vi "摩擦力F.vi"(8 "计算参数 in":T2, 9 "输入参数":T1, 10 "进油口压力数组 in":dbl[](array[numeric]), 11 "行程数组 in":dbl[](array[numeric])) -> (0 "计算参数 out":T2, 2 "进油口压力数组 out":dbl[](array[numeric]), 3 "行程数组 out":dbl[](array[numeric]))   [LabVIEW 2013]
doc: "此程序计算开启关闭时间\nCL=tv2-tv1\nOP=ts2-ts1"
panel:
  out "P":dbl[](array[numeric])
  out "TIME_DOWN":dbl[](array[numeric])
  out "TIME_UP":dbl[](array[numeric])
  out "V":dbl[](array[numeric])
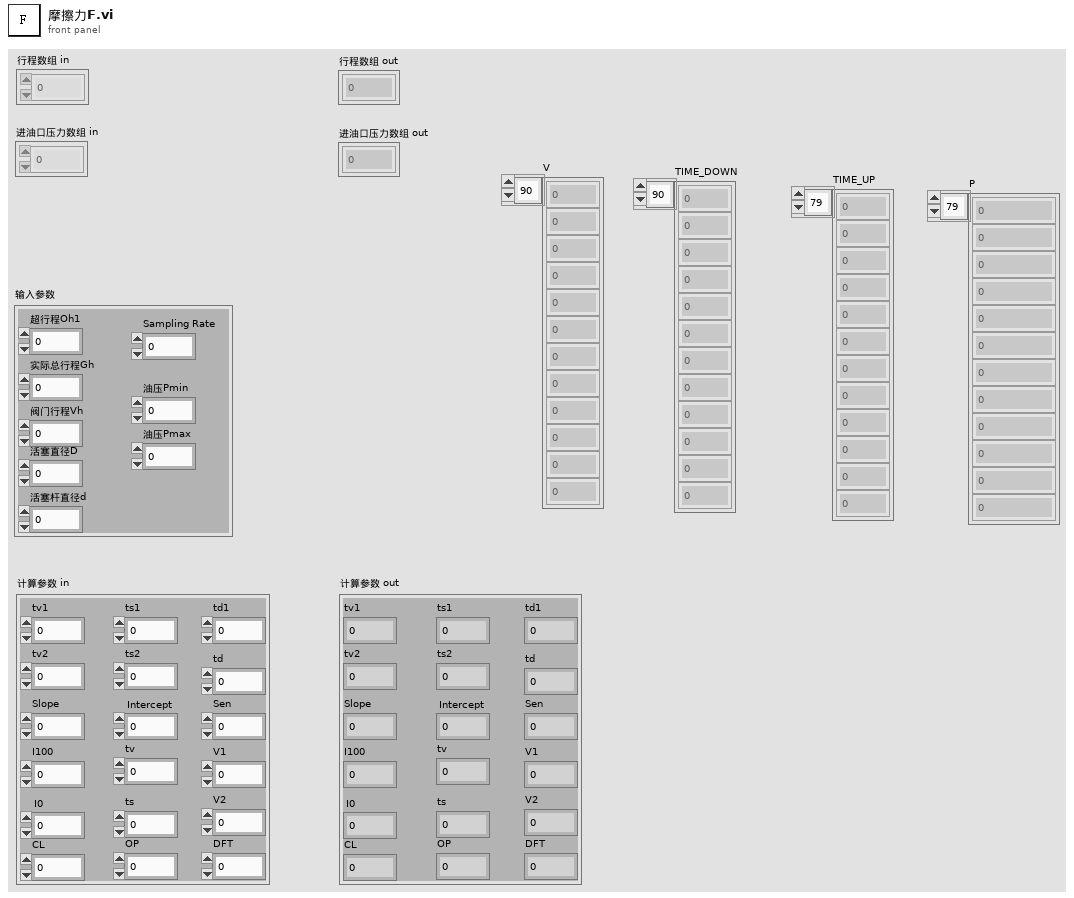
[diagram p1: front panel]
types:
  T1 = cluster{"超行程Oh1":dbl, "实际总行程Gh":dbl, "阀门行程Vh":dbl, "活塞直径D":dbl, "活塞杆直径d":dbl, "油压Pmin":dbl, "油压Pmax":dbl, "Sampling Rate":dbl}
  T2 = cluster{"tv1":dbl, "tv2":dbl, "tv":dbl, "ts1":dbl, "ts2":dbl, "ts":dbl, "td1":dbl, "td":dbl, "Slope":dbl, "Intercept":dbl, "I100":dbl, "I0":dbl, "Sen":dbl, "V1":dbl, "V2":dbl, "CL":dbl, "OP":dbl, "DFT":dbl}
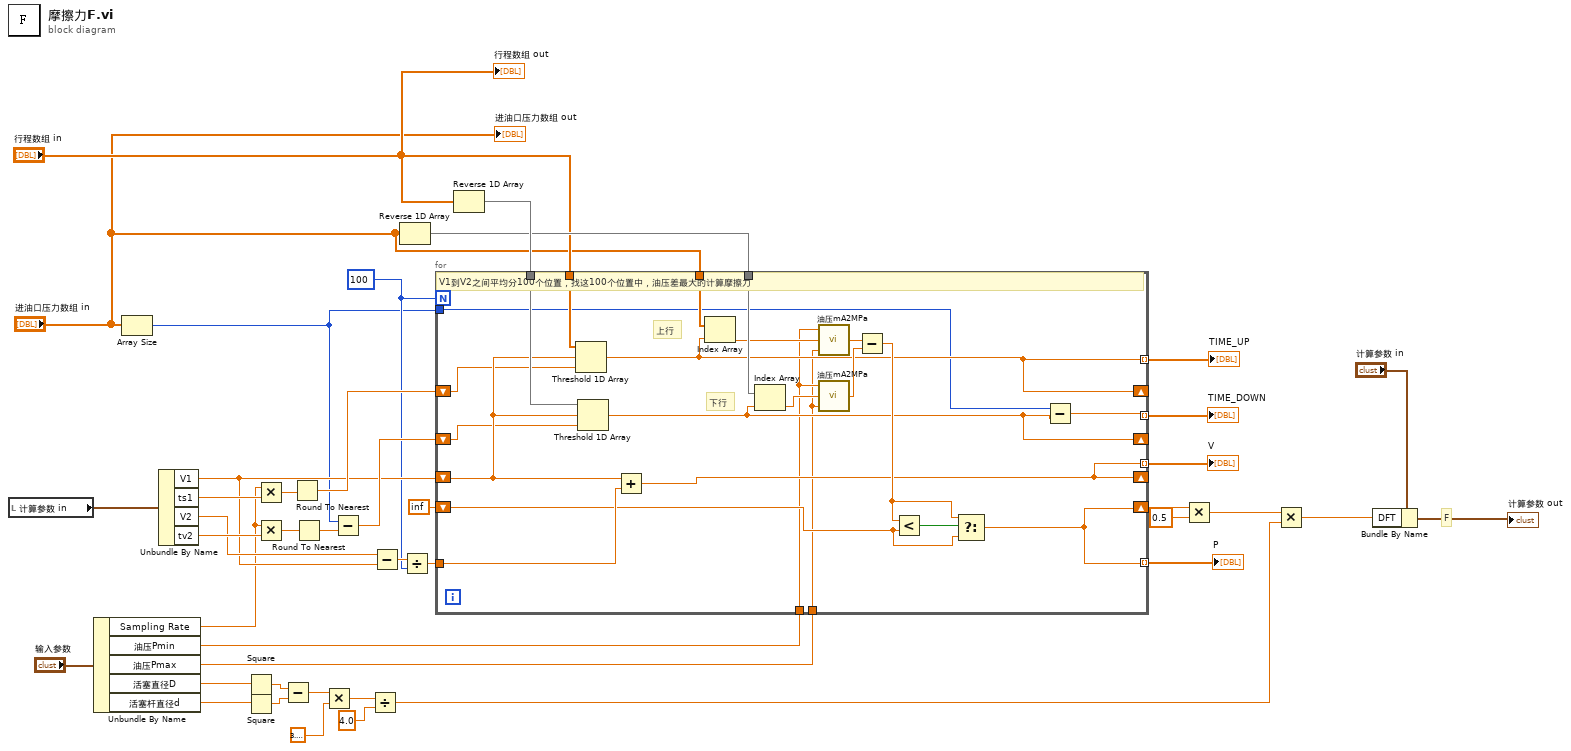
[diagram p0: block diagram]
diagram:
  w20 = 100
  # "F"
  n1 = local read "计算参数 in"() -> (w40:T2)
  n2 = Unbundle By Name("输入参数") -> ("Sampling Rate"=w1:dbl, "油压Pmin"=w3:dbl, "油压Pmax"=w2:dbl, "活塞直径D"=w38:dbl, "活塞杆直径d"=w37:dbl)
  n3 = Array Size(array="进油口压力数组 in") -> (size(s)=w5:i32)
  n4 = Unbundle By Name(w40) -> ("V1"=w22:dbl, "ts1"=w29:dbl, "V2"=w23:dbl, "tv2"=w27:dbl)
  n5 = Square(x=w38) -> (x^2=w36:dbl)
  n6 = Square(x=w37) -> (x^2=w35:dbl)
  n7 = Multiply(x=w1, y=w29) -> (x*y=w30:dbl)
  n8 = Multiply(x=w1, y=w27) -> (x*y=w28:dbl)
  n9 = Subtract(x=w36, y=w35) -> (x-y=w34:dbl)
  n10 = Round To Nearest(number=w30) -> (nearest integer value=w25:dbl)
  n11 = Round To Nearest(number=w28) -> (nearest integer value=w26:dbl)
  n12 = Multiply(x=w34, y=3.141592653589793) -> (x*y=w32:dbl)
  n13 = Subtract(x=w5, y=w26) -> (x-y=w24:dbl)
  n14 = Divide(x=w32, y=4.0) -> (x/y=w13:dbl)
  n15 = Subtract(x=w23, y=w22) -> (x-y=w21:dbl)
  n16 = Reverse 1D Array(array="进油口压力数组 in") -> (reversed array=w16:dbl[])
  n17 = Divide(x=w21, y=w20) -> (x/y=w19:dbl)
  n18 = Reverse 1D Array(array="行程数组 in") -> (reversed array=w17:dbl[])
  n19 = for {
    N: w20 -> [_]
    shift-right: [w49] -> _
    shift-left: w25 -> [w60]
    shift-right: [w47] -> _
    shift-left: w24 -> [w61]
    tunnel: "行程数组 in" -> [w65]
    shift-right: [w50] -> _
    shift-left: w22 -> [w62]
    tunnel: w19 -> [w64]
    shift-right: [w45] -> w15
    shift-left: inf -> [w56]
    tunnel: w17 -> [w63]
    tunnel: w16 -> [w59]
    tunnel: "进油口压力数组 in" -> [w58]
    tunnel: [w50] -> w8 mode=indexing
    tunnel: [w49] -> w7 mode=indexing
    tunnel: [w48] -> w6 mode=indexing
    tunnel: w5 -> [w46]
    tunnel: [w45] -> w4 mode=indexing
    tunnel: w3 -> [w44]
    tunnel: w2 -> [w43]
    # "下行"
    # "上行"
    # "V1到V2之间平均分100个位置，找这100个位置中，油压差最大的计算摩擦力"
    n20 = Threshold 1D Array(1:w60, 2:w62, 3:w65) -> (0:w49:dbl)
    n21 = Threshold 1D Array(1:w61, 2:w62, 3:w63) -> (0:w47:dbl)
    n22 = Add(x=w62, y=w64) -> (x+y=w50:dbl)
    n23 = Index Array(array=w58, index=w49) -> (element=w53:dbl)
    n24 = Index Array(array=w59, index=w47) -> (element=w52:dbl)
    n25 = call "油压mA2MPa.vi"("油压Max"=w43, "油压mA"=w53, "油压Min"=w44) -> ("油压MPa"=w54:dbl)  [unwired: 2 in]
    n26 = call "油压mA2MPa.vi"("油压Max"=w43, "油压mA"=w52, "油压Min"=w44) -> ("油压MPa"=w51:dbl)  [unwired: 2 in]
    n27 = Subtract(x=w54, y=w51) -> (x-y=w55:dbl)
    n28 = Less?(x=w55, y=w56) -> (x < y?=w57:bool)
    n29 = Select(t=w55, s=w57, f=w56) -> (s? t:f=w45:dbl)
    n30 = Subtract(x=w46, y=w47) -> (x-y=w48:dbl)
  }
  "V" <- w8
  "TIME_UP" <- w7
  "TIME_DOWN" <- w6
  "P" <- w4
  n31 = Multiply(x=w15, y=0.5) -> (x*y=w9:dbl)
  n32 = Multiply(x=w9, y=w13) -> (x*y=w12:dbl)
  n33 = Bundle By Name(cluster="计算参数 in", "DFT"=w12) -> (→"计算参数 out":T2)
  "进油口压力数组 out" <- "进油口压力数组 in"
  "行程数组 out" <- "行程数组 in"
